vi "Build Notifier Controller.vi"(4 "Paras In 2":variant, 6 "Paras In":variant, 7 "Node Controller Factory in":refnum<class "Node Controller Factory.lvclass">, 8 "error in (no error)":errorcluster, 9 "Notifier Type":refnum<class "Notifier.lvclass">, 10 "System Actors In":refnum<class "System Actor.lvclass">[](array[class]), 11 "Root Actor In":refnum<class "Root Actor.lvclass">) -> (0 "error out":errorcluster, 2 "System Actors Out":refnum<class "System Actor.lvclass">[](array[class]), 3 "Root Actor Out":refnum<class "Root Actor.lvclass">, 5 "Node Controller Factory out":refnum<class "Node Controller Factory.lvclass">)   [LabVIEW 2024, in "Node Controller Factory.lvclass"]
uses:
  Node Controller Factory.lvclass
  Actor/Root Actor/Root Actor.lvclass
  Actor/System Actor/System Actor.lvclass
  Actor Assistant/Notifier/Notifier.lvclass
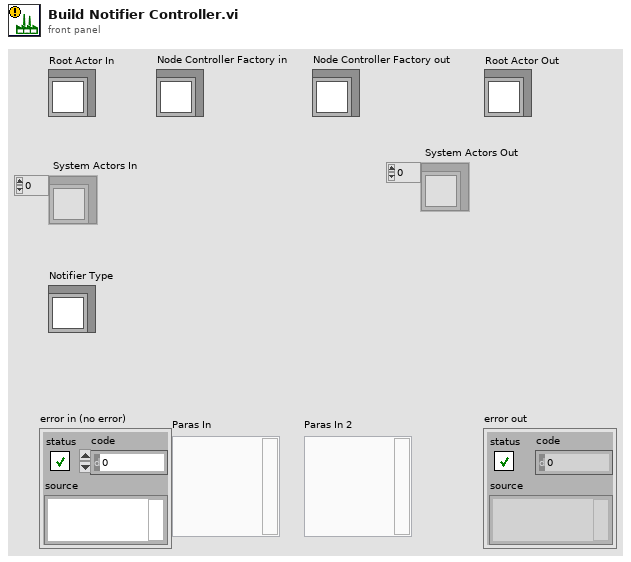
[diagram p1: front panel]
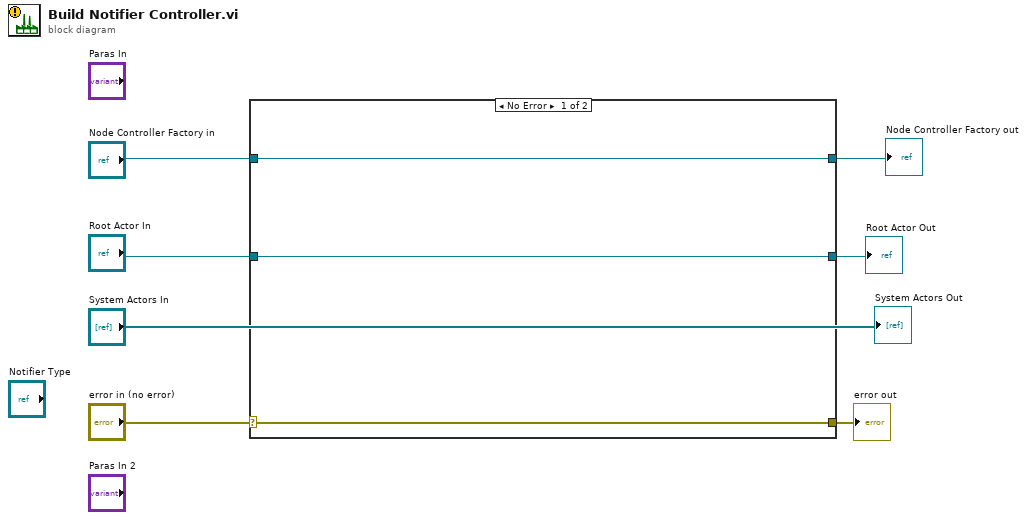
[diagram p0: block diagram]
diagram:
  n1 = case shown="No Error" "error in (no error)" {
    selector: "error in (no error)" -> [w9 w13]
    tunnel: [w9 w13] -> w6
    tunnel: [w10 w12] -> w2
    tunnel: "Node Controller Factory in" -> [w10 w12]
    tunnel: [w8 w11] -> w4
    tunnel: "Root Actor In" -> [w8 w11]
    frame No Error {
    }
    frame Error {
    }
  }
  "Node Controller Factory out" <- w2
  "error out" <- w6
  "Root Actor Out" <- w4
  "System Actors Out" <- "System Actors In"
